vi "Aufgabe1.vi"   [LabVIEW 2016]
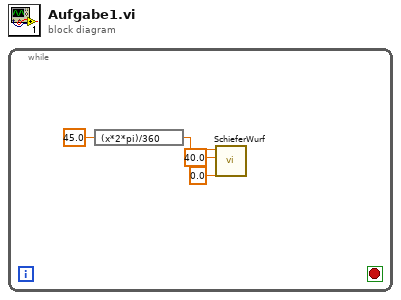
[diagram p0: block diagram]
diagram:
  n1 = while {
    stop <- _ stop-if-true
    n2 = expression code="(x*2*pi)/360"(45.0) -> (w4:dbl)
    n3 = call "SchieferWurf.vi"("t [s]"=0.0, "v0 [m/s]"=40.0, "alpha [rad]"=w4) -> ()  [unwired: 7 in, 2 out]
  }
